vi "Queue Comms Dequeue.vi"(8 "error in (no error)":errorcluster, 11 "queue In":refnum<queue>) -> (0 "error out":errorcluster, 3 "Element":T1)   [LabVIEW 2020, in "Error Handler.lvlib"]
uses:
  Error Handler.lvlib
  Private Controls/Element.ctl
  Private Controls/Module Action.ctl
  Queue FGV Action.ctl
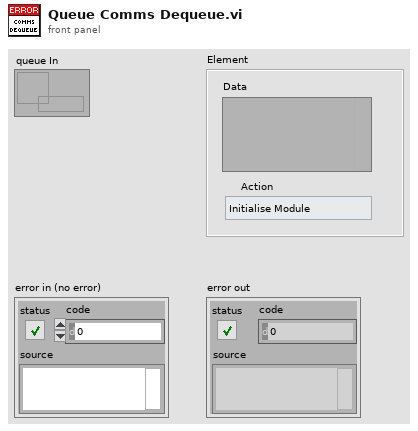
[diagram p1: front panel]
types:
  T1 = typedef "Error Handler.lvlib/Element.ctl" = cluster{"Action":T2, "Data":variant}
  T2 = typedef "Error Handler.lvlib/Module Action.ctl" = enum16{"Initialise Module", "Modify Reaction to Error", "Log to File", "Prompt User", "External Error", "Internal Error", "Exit"}
  T3 = typedef "Error Handler.lvlib/Queue FGV Action.ctl" = enum16{"Get", "Set", "Release"}
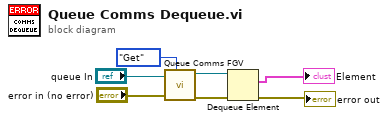
[diagram p0: block diagram]
diagram:
  n1 = call "Queue Comms FGV.vi"("Action"=Queue_FGV_Action."Get", "error in (no error)"="error in (no error)", "queue In"="queue In") -> ("error out"=w6:errorcluster, "queue In"=w7:refnum<queue>)  [unwired: 7 in]
  n2 = Dequeue Element(queue=w7, error in (no error)=w6) -> (element=→"Element":T1, error out=→"error out":errorcluster)  [unwired: 1 in, 2 out]
